vi "FIFOFileObject.vi"(1 ".sm file format":bool, 2 "function (open:0)":enum16{"open", "write", "close"}(ring), 3 "error in (no error)":errorcluster, 4 "count":u32, 5 "buffer":u32[](array[numeric]), 6 "Destination:":path) -> (0 "error out":errorcluster)   [LabVIEW 2009]
panel:
  in  "Column Definitions 2":T1(array[cluster])=[{"Column Name"="Time High", "Resolution"=214.74836475, "Offset"=0.0, "Channel Names"=[]}, {"Column Name"="Time Low", "Resolution"=5e-08, "Offset"=0.0, "Channel Names"=[]}, {"Column Name"="Channel", "Resolution"=0.0, "Offset"=0.0, "Channel Names"=["L1D1", "L1D2", "L1D3", "L1D4", "L2D1", "L2D2", "L2D3", "L2D4", "L3D1", "L3D2", "L3D3", "L3D4", "L4D1", "L4D2", "L4D3", "L4D4"]}] {"Offset" format="%.2f"; "Resolution" format="%.5e"}
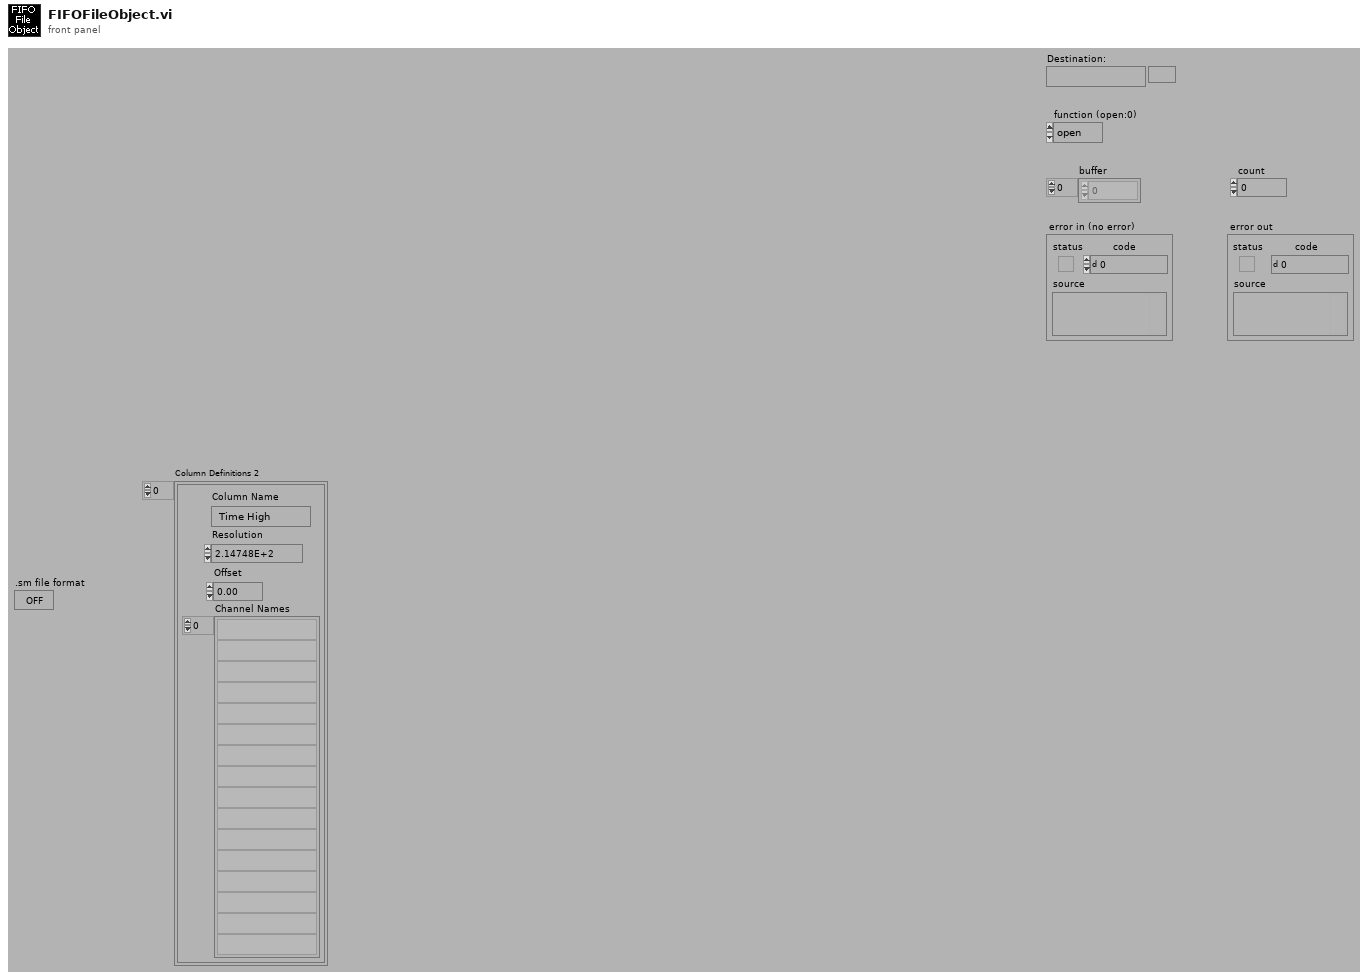
[diagram p1: front panel]
types:
  T1 = cluster{"Column Name":string, "Resolution":dbl, "Offset":dbl, "Channel Names":string[]}[]
  T2 = enum16{"open", "open or create", "create or replace", "create", "open (read only)"}
  T3 = cluster{"router channels":u8[], "macro times(50ns steps)":u32[], "micro times":u16[], "invalid times":u32[], "gap times":u32[]}
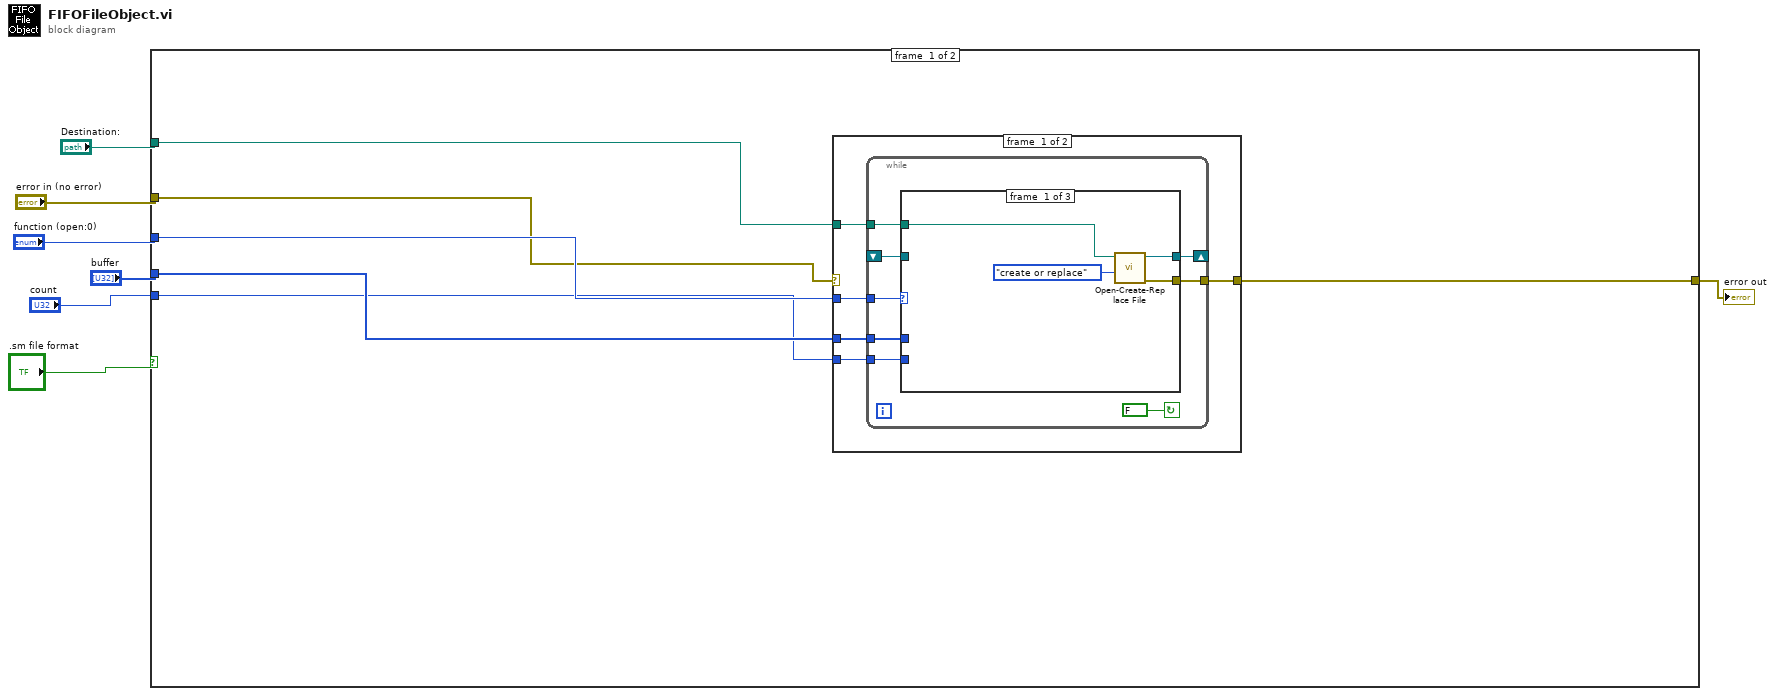
[diagram p0: block diagram]
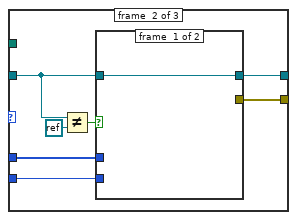
[diagram p2: hidden frame]
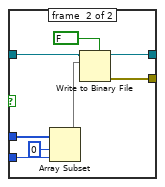
[diagram p3: hidden frame]
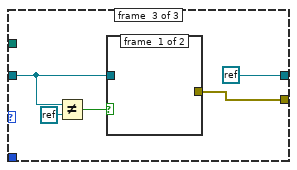
[diagram p4: hidden frame]
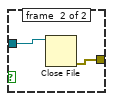
[diagram p5: hidden frame]
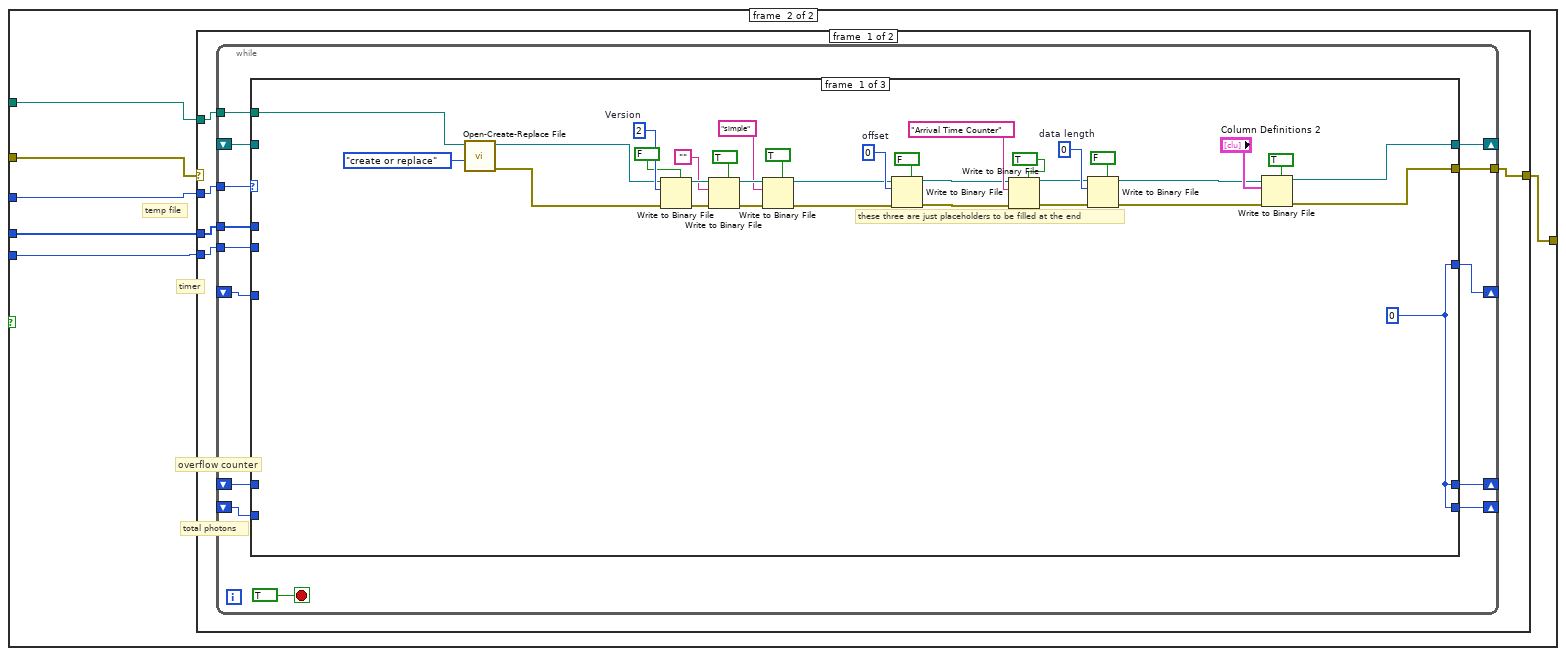
[diagram p7: hidden frame]
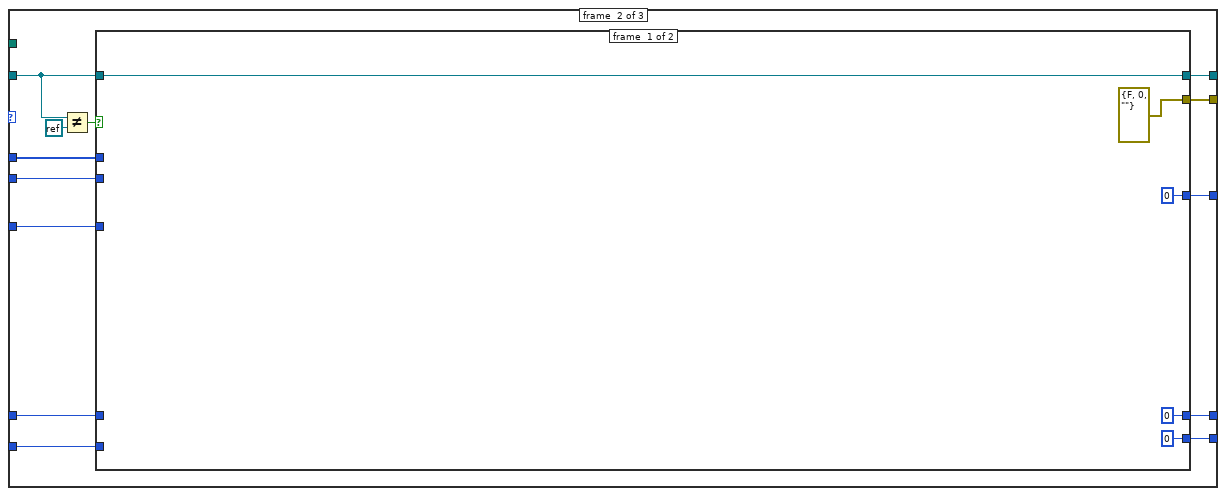
[diagram p8: hidden frame]
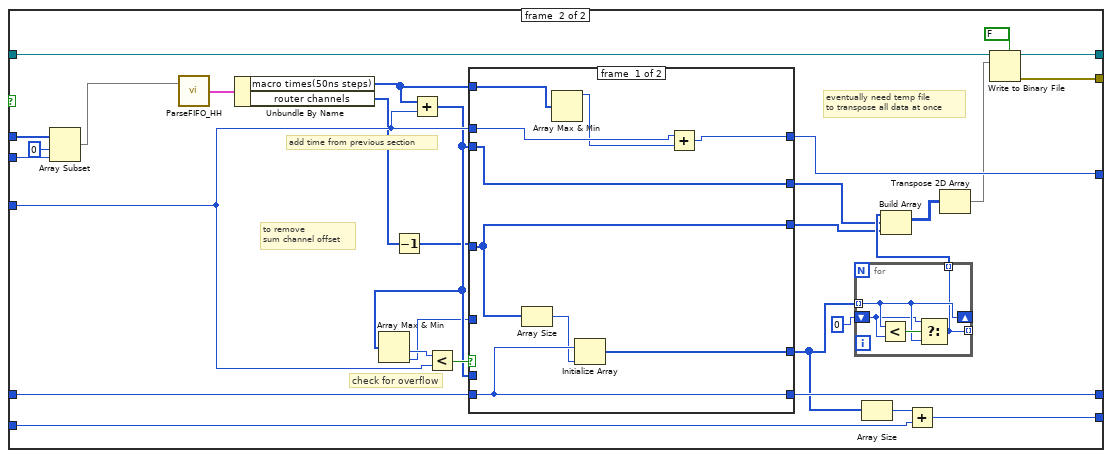
[diagram p9: hidden frame]
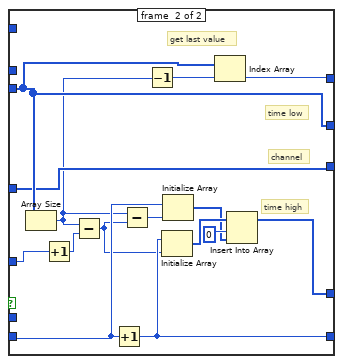
[diagram p10: hidden frame]
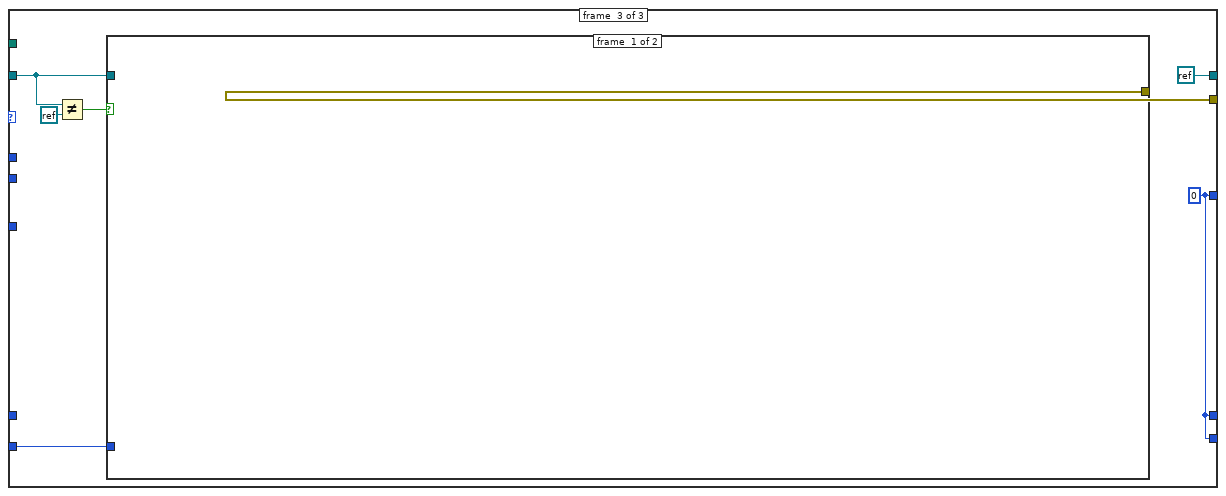
[diagram p11: hidden frame]
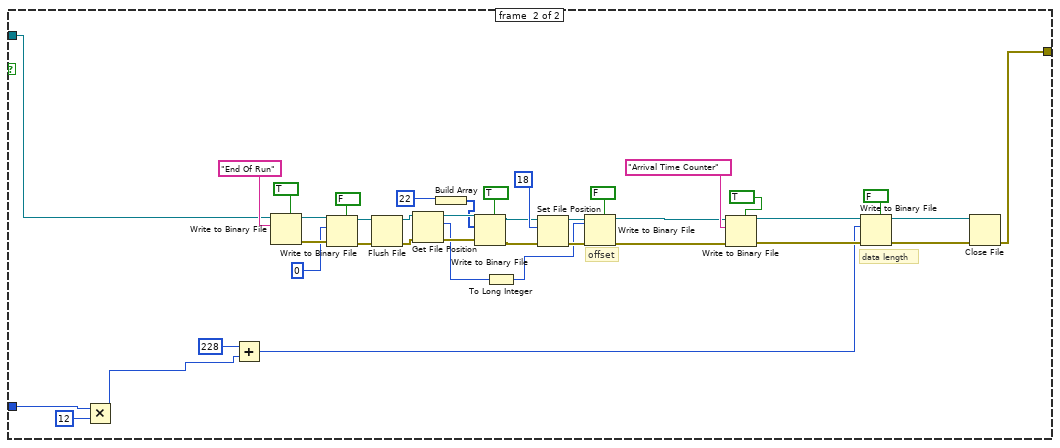
[diagram p12: hidden frame]
diagram:
  n1 = case shown="True" ".sm file format" {
    tunnel: "buffer" -> [w13 w57]
    tunnel: "function (open:0)" -> [w12 w59]
    tunnel: "error in (no error)" -> [w11 w60]
    tunnel: "Destination:" -> [w10 w58]
    tunnel: "count" -> [w9 w56]
    tunnel: [w8 w55] -> w1
    frame #0 {
      n2 = case shown="No Error" w11 {
        selector: w11 -> [_ w54]
        tunnel: w10 -> [w18 _]
        tunnel: [w17 w54] -> w8
        tunnel: w12 -> [w16 _]
        tunnel: w9 -> [w15 _]
        tunnel: w13 -> [w14 _]
        frame #0 {
          n3 = while {
            tunnel: w18 -> [w25]
            tunnel: [w24] -> w17
            shift-right: [w23] -> _
            shift-left: _ -> [w22]
            tunnel: w16 -> [w21]
            tunnel: w15 -> [w20]
            tunnel: w14 -> [w19]
            stop <- FALSE continue-if-true
            n4 = case shown="\"write\", Default" w21 {
              tunnel: w25 -> [w27 _ _]
              tunnel: [w29 w34 w50] -> w24
              tunnel: [w28 w37 refnum<k0> refnum] -> w23
              tunnel: w22 -> [_ w31 w48]
              tunnel: w20 -> [_ w36 _]
              tunnel: w19 -> [_ w35 _]
              frame #0 {
                n5 = call "Open-Create-Replace File.vi"("function (open:0)"=T2."create or replace", "file path"=w27) -> ("error out"=w29:errorcluster, "refnum"=w28:refnum<file>)  [unwired: 6 in, 2 out]
              }
              frame #1 {
                n6 = Not Equal?(x=w31, y=refnum<k0> refnum) -> (x != y?=w33:bool)
                n7 = case shown="True" w33 {
                  tunnel: [w38 w44] -> w37
                  tunnel: w36 -> [_ w43]
                  tunnel: w35 -> [_ w42]
                  tunnel: [_ w41] -> w34
                  tunnel: w31 -> [w38 w40]
                  frame #0 {
                  }
                  frame #1 {
                    n8 = Array Subset(array=w42, index=0, length=w43) -> (w45:u32[])
                    n9 = Write to Binary File(file (use dialog)=w40, data=w45, 5:FALSE ("prepend array or string size? (T)")) -> (refnum out=w44:refnum<file>, error out=w41:errorcluster)  [unwired: 3 in, 1 out]
                  }
                }
              }
              frame #2 {
                n10 = Not Equal?(x=w48, y=refnum<k0> refnum) -> (x != y?=w47:bool)
                n11 = case shown="True" w47 {
                  tunnel: [_ w53] -> w50
                  tunnel: w48 -> [_ w52]
                  frame #0 {
                  }
                  frame #1 {
                    n12 = Close File(refnum=w52) -> (error out=w53:errorcluster)  [unwired: 1 in, 1 out]
                  }
                }
              }
            }
          }
        }
        frame #1 {
        }
      }
    }
    frame #1 {
      # "temp file"
      # "total photons"
      # "overflow counter"
      # "timer"
      n13 = case shown="No Error" w60 {
        selector: w60 -> [_ w235]
        tunnel: w58 -> [w65 _]
        tunnel: [w64 w235] -> w55
        tunnel: w59 -> [w63 _]
        tunnel: w56 -> [w62 _]
        tunnel: w57 -> [w61 _]
        frame #0 {
          n14 = while {
            tunnel: w65 -> [w78]
            tunnel: [w77] -> w64
            shift-right: [w76] -> _
            shift-left: _ -> [w75]
            tunnel: w63 -> [w74]
            tunnel: w62 -> [w73]
            tunnel: w61 -> [w72]
            shift-right: [w71] -> _
            shift-left: _ -> [w70]
            shift-right: [w69] -> _
            shift-left: _ -> [w68]
            shift-right: [w67] -> _
            shift-left: _ -> [w66]
            stop <- TRUE stop-if-true
            n15 = case shown="\"open\"" w74 {
              tunnel: w78 -> [w111 _ _]
              tunnel: [w84 w114 w195] -> w77
              tunnel: [w83 w125 refnum<k0> refnum] -> w76
              tunnel: w75 -> [_ w113 w193]
              tunnel: w73 -> [_ w124 _]
              tunnel: w72 -> [_ w123 _]
              tunnel: [w82 w120 w191] -> w71
              tunnel: w70 -> [_ w119 _]
              tunnel: [w82 w118 w191] -> w69
              tunnel: w68 -> [_ w117 _]
              tunnel: [w82 w116 w191] -> w67
              tunnel: w66 -> [_ w115 w190]
              frame #0 {
                w87 = 0  # data length
                w97 = 0  # offset
                w110 = 2  # Version
                w82 = u32 0
                # "these three are just placeholders to be filled at the end"
                n16 = call "Open-Create-Replace File.vi"("function (open:0)"=T2."create or replace", "file path"=w111) -> ("error out"=w95:errorcluster, "refnum"=w94:refnum<file>)  [unwired: 6 in, 2 out]
                n17 = Write to Binary File(file (use dialog)=w94, data=w110, error in=w95, 5:FALSE ("prepend array or string size? (T)")) -> (refnum out=w109:refnum<file>, error out=w105:errorcluster)  [unwired: 2 in, 1 out]
                n18 = Write to Binary File(file (use dialog)=w109, data="", error in=w105, 5:TRUE ("prepend array or string size? (T)")) -> (refnum out=w107:refnum<file>, error out=w104:errorcluster)  [unwired: 2 in, 1 out]
                n19 = Write to Binary File(file (use dialog)=w107, data="simple", error in=w104, 5:TRUE ("prepend array or string size? (T)")) -> (refnum out=w81:refnum<file>, error out=w80:errorcluster)  [unwired: 2 in, 1 out]
                n20 = Write to Binary File(file (use dialog)=w81, data=w97, error in=w80, 5:FALSE ("prepend array or string size? (T)")) -> (refnum out=w99:refnum<file>, error out=w98:errorcluster)  [unwired: 2 in, 1 out]
                n21 = Write to Binary File(file (use dialog)=w99, data="Arrival Time Counter", error in=w98, 5:TRUE ("prepend array or string size? (T)")) -> (refnum out=w86:refnum<file>, error out=w85:errorcluster)  [unwired: 2 in, 1 out]
                n22 = Write to Binary File(file (use dialog)=w86, data=w87, error in=w85, 5:FALSE ("prepend array or string size? (T)")) -> (refnum out=w89:refnum<file>, error out=w88:errorcluster)  [unwired: 2 in, 1 out]
                n23 = Write to Binary File(file (use dialog)=w89, data="Column Definitions 2", error in=w88, 5:TRUE ("prepend array or string size? (T)")) -> (refnum out=w83:refnum<file>, error out=w84:errorcluster)  [unwired: 2 in, 1 out]
              }
              frame #1 {
                n24 = Not Equal?(x=w113, y=refnum<k0> refnum) -> (x != y?=w122:bool)
                n25 = case shown="True" w122 {
                  tunnel: [w130 w133] -> w125
                  tunnel: w124 -> [_ w159]
                  tunnel: w123 -> [_ w158]
                  tunnel: w113 -> [w130 w134]
                  tunnel: [u32 0 w153] -> w120
                  tunnel: w119 -> [_ w152]
                  tunnel: [u32 0 w151] -> w118
                  tunnel: w117 -> [_ w150]
                  tunnel: [0 w141] -> w116
                  tunnel: w115 -> [_ w140]
                  tunnel: [errorcluster {"status"=FALSE, "code"=0, "source"=""} ("error out") w139] -> w114
                  frame #0 {
                  }
                  frame #1 {
                    # "eventually need temp file\nto transpose all data at once"
                    # "to remove \nsum channel offset"
                    # "check for overflow"
                    # "add time from previous section"
                    n26 = Array Subset(array=w158, index=0, length=w159) -> (w136:u32[])
                    n27 = call "ParseFIFO_HH.vi"("RawData"=w136) -> ("RawData Out"=w149:T3)  [unwired: 1 in]
                    n28 = Unbundle By Name(w149) -> ("macro times(50ns steps)"=w137:u32[], "router channels"=w145:u8[])
                    n29 = Decrement(x=w145) -> (x-1=w146:u8[])
                    n30 = Add(x=w137, y=w150) -> (x+y=w147:u32[])
                    n31 = Array Max & Min(array=w147) -> (min value=w144:u32, min index (indices)=w143:i32)  [unwired: 2 out]
                    n32 = Less?(x=w144, y=w150) -> (x < y?=w148:bool)
                    n33 = case shown="False" w148 {
                      tunnel: w147 -> [_ _]
                      tunnel: [w166 w184] -> w151
                      tunnel: [w163 w173] -> w155
                      tunnel: [w162 w172] -> w154
                      tunnel: w147 -> [w163 w173]
                      tunnel: w146 -> [w162 w172]
                      tunnel: w152 -> [w169 w183]
                      tunnel: [w169 w182] -> w153
                      tunnel: [w161 w170] -> w135
                      tunnel: w150 -> [w168 _]
                      tunnel: w137 -> [w164 _]
                      tunnel: w143 -> [_ w179]
                      frame #0 {
                        n34 = Array Size(array=w162) -> (size(s)=w167:i32)
                        n35 = Array Max & Min(array=w164) -> (max value=w165:u32)  [unwired: 3 out]
                        n36 = Initialize Array(w169, w167) -> (w161:u32[])
                        n37 = Add(x=w168, y=w165) -> (x+y=w166:u32)
                      }
                      frame #1 {
                        # "time high"
                        # "channel"
                        # "time low"
                        # "get last value"
                        n38 = Array Size(array=w173) -> (size(s)=w171:i32)
                        n39 = Increment(x=w179) -> (x+1=w178:i32)
                        n40 = Subtract(x=w171, y=w178) -> (x-y=w176:i32)
                        n41 = Increment(x=w183) -> (x+1=w182:u32)
                        n42 = Subtract(x=w171, y=w176) -> (x-y=w177:i32)
                        n43 = Decrement(x=w171) -> (x-1=w180:i32)
                        n44 = Initialize Array(w182, w176) -> (w175:u32[])
                        n45 = Initialize Array(w183, w177) -> (w174:u32[])
                        n46 = Index Array(array=w173, index=w180) -> (element=w184:u32)
                        n47 = Insert Into Array(array=w175, index=0, new element=w174) -> (w170:u32[])
                      }
                    }
                    n48 = for {
                      tunnel: w135 -> [w187] mode=indexing
                      shift-right: [w187] -> _
                      shift-left: 0 ("x") -> [w186]
                      tunnel: [w185] -> _ mode=indexing
                      tunnel: [w185] -> w157 mode=indexing
                      n49 = Less?(x=w187, y=w186) -> (x < y?=w188:bool)
                      n50 = Select(t=w186, s=w188, f=w187) -> (s? t:f=w185:u32)
                    }
                    n51 = Array Size(array=w135) -> (size(s)=w142:i32)
                    n52 = Build Array(w157, w155, w154) -> (w132:u32[][])
                    n53 = Add(x=w142, y=w140) -> (x+y=w141:u32)
                    n54 = Transpose 2D Array(2D array=w132) -> (transposed array=w131:u32[][])
                    n55 = Write to Binary File(file (use dialog)=w134, data=w131, 5:FALSE ("prepend array or string size? (T)")) -> (refnum out=w133:refnum<file>, error out=w139:errorcluster)  [unwired: 3 in, 1 out]
                  }
                }
              }
              frame #2 {
                w191 = u32 0
                n56 = Not Equal?(x=w193, y=refnum<k0> refnum) -> (x != y?=w192:bool)
                n57 = case shown="True" w192 {
                  tunnel: [_ w211] -> w195
                  tunnel: w193 -> [_ w203]
                  tunnel: w190 -> [_ w210]
                  frame #0 {
                  }
                  frame #1 {
                    # "data length"
                    # "offset"
                    n58 = Multiply(x=w210, y=u32 12) -> (x*y=w198:u32)
                    n59 = Add(x=u32 228, y=w198) -> (x+y=w197:u32)
                    n60 = Write to Binary File(file (use dialog)=w203, data="End Of Run", 5:TRUE ("prepend array or string size? (T)")) -> (refnum out=w225:refnum<file>, error out=w224:errorcluster)  [unwired: 3 in, 1 out]
                    n61 = Write to Binary File(file (use dialog)=w225, data=0, error in=w224, 5:FALSE ("prepend array or string size? (T)")) -> (refnum out=w221:refnum<file>, error out=w220:errorcluster)  [unwired: 2 in, 1 out]
                    n62 = Flush File(refnum=w221, error in=w220) -> (refnum out=w219:refnum<file>, error out=w218:errorcluster)
                    n63 = Get File Position(4:w218, 7:w219) -> (0:w230:errorcluster, 2:w214:i64, 3:w229:refnum<file>)
                    n64 = Build Array(22) -> (w216:i32[])
                    n65 = Write to Binary File(file (use dialog)=w229, data=w216, error in=w230, 5:TRUE ("prepend array or string size? (T)")) -> (refnum out=w227:refnum<file>, error out=w226:errorcluster)  [unwired: 2 in, 1 out]
                    n66 = To Long Integer(number=w214) -> (32bit integer=w228:i32)
                    n67 = Set File Position(offset (in bytes) (0)=18, refnum=w227, error in=w226) -> (refnum out=w233:refnum<file>, error out=w232:errorcluster)  [unwired: 1 in]
                    n68 = Write to Binary File(file (use dialog)=w233, data=w228, error in=w232, 5:FALSE ("prepend array or string size? (T)")) -> (refnum out=w200:refnum<file>, error out=w199:errorcluster)  [unwired: 2 in, 1 out]
                    n69 = Write to Binary File(file (use dialog)=w200, data="Arrival Time Counter", error in=w199, 5:TRUE ("prepend array or string size? (T)")) -> (refnum out=w205:refnum<file>, error out=w204:errorcluster)  [unwired: 2 in, 1 out]
                    n70 = Write to Binary File(file (use dialog)=w205, data=w197, error in=w204, 5:FALSE ("prepend array or string size? (T)")) -> (refnum out=w201:refnum<file>, error out=w202:errorcluster)  [unwired: 2 in, 1 out]
                    n71 = Close File(refnum=w201, error in=w202) -> (error out=w211:errorcluster)  [unwired: 1 out]
                  }
                }
              }
            }
          }
        }
        frame #1 {
        }
      }
    }
  }
  "error out" <- w1
